vi "Initialize_Angle.vi"(8 "error in (no error)":errorcluster, 9 "Radius":dbl, 10 "Angle.lvclass":refnum<class "Angle.lvclass">) -> (0 "error out":errorcluster, 3 "PolarVector out":refnum<class "PolarVector.lvclass">)   [LabVIEW 2013, in "PolarVector.lvclass"]
doc: "Takes in a DBL radius and an Angle object and converts it to a PolarVector object."
uses:
  PolarVector.lvclass
  Angles/Angle/Angle.lvclass
  PolarVector.lvclass/PolarVector.ctl
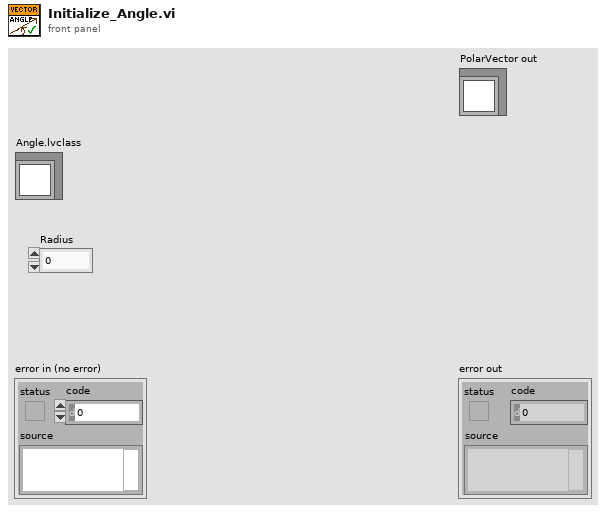
[diagram p1: front panel]
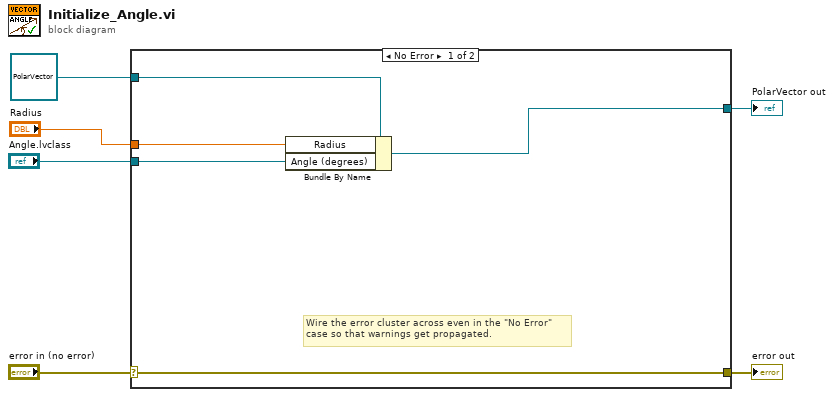
[diagram p0: block diagram]
diagram:
  n1 = case shown="No Error" "error in (no error)" {
    selector: "error in (no error)" -> [w8 w13]
    tunnel: [w8 w13] -> w5
    tunnel: [w10 w12] -> w1
    tunnel: "Angle.lvclass" -> [w11 _]
    tunnel: "Radius" -> [w9 _]
    tunnel: refnum<class "PolarVector.lvclass"> refnum ("PolarVector out") -> [w7 w12]
    frame No Error {
      # "Wire the error cluster across even in the \"No Error\"\ncase so that warnings get propagated."
      n2 = Bundle By Name(cluster=w7, "Radius"=w9, "Angle (degrees)"=w11) -> (w10:refnum<class "PolarVector.lvclass">)
    }
    frame Error {
    }
  }
  "error out" <- w5
  "PolarVector out" <- w1
